vi "2.vi"() -> ()   [LabVIEW 2017]
panel:
  out "波形图":dbl[](graph)
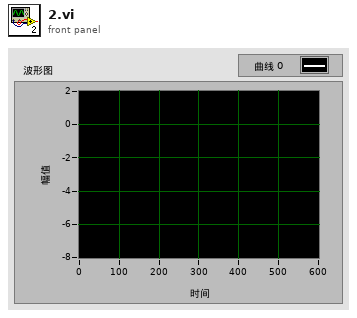
[diagram p1: front panel]
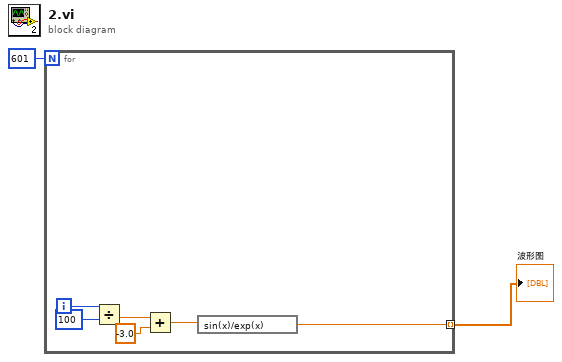
[diagram p0: block diagram]
diagram:
  n1 = for {
    N: 601 -> [_]
    tunnel: [w3] -> w1 mode=indexing
    i -> [w8]
    n2 = Divide(x=w8, y=100) -> (x/y=w6:dbl)
    n3 = Add(x=w6, y=-3.0) -> (x+y=w4:dbl)
    n4 = expression code="sin(x)/exp(x)"(w4) -> (w3:dbl)
  }
  "波形图" <- w1
